vi "Set NotifyIcon Tip Text.vi"(4 "error in (no error)":errorcluster, 6 "Icon Tip Text":string, 7 "NotifyIcon":refnum<k24>) -> (0 "error out":errorcluster, 3 "NotifyIcon out":refnum<k24>)   [LabVIEW 2014, in "NotifyIcon.lvlib"]
uses:
  NotifyIcon.lvlib
  System.Windows.Forms
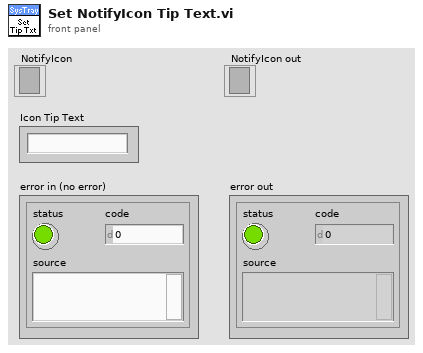
[diagram p1: front panel]
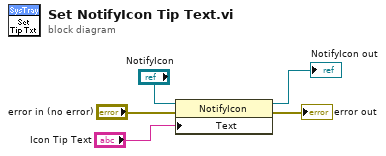
[diagram p0: block diagram]
diagram:
  n1 = property class="NotifyIcon"(reference="NotifyIcon", error in="error in (no error)", "Text"="Icon Tip Text") -> (reference out=→"NotifyIcon out":refnum<k24>, error out=→"error out":errorcluster)
